vi "Create Custom Error Handler.vi"(5 "Error Description":string, 6 "T: Warning":bool, 7 "code":i32, 8 "error in":errorcluster, 10 "F: Create Error":bool=TRUE, 11 "T: Create Error":bool) -> (0 "error out":errorcluster)   [LabVIEW 2019, in "MView.lvlib"]
uses:
  Lib.llb/MView.lvlib
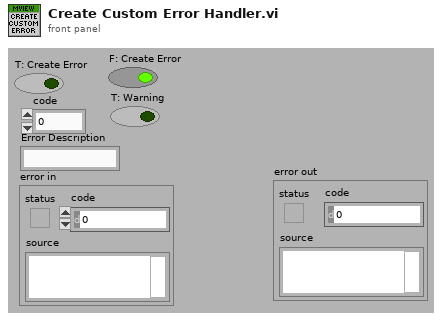
[diagram p1: front panel]
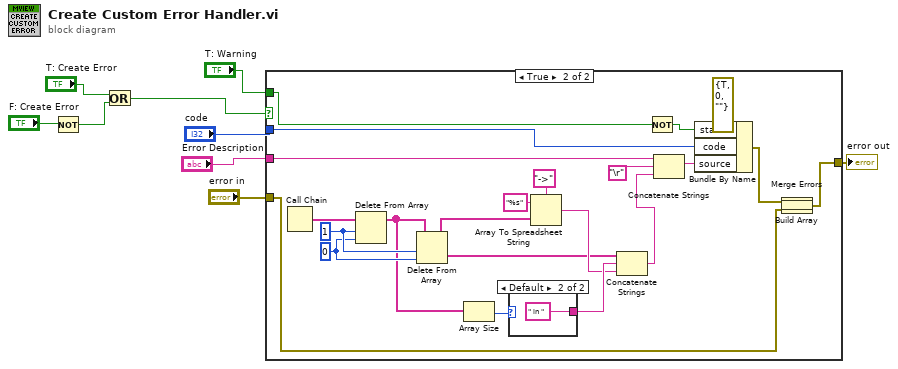
[diagram p0: block diagram]
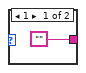
[diagram p3: hidden frame]
diagram:
  n1 = Not(x="F: Create Error") -> (.not. x?=w2:bool)
  n2 = Or(x="T: Create Error", y=w2) -> (x .or. y?=w1:bool)
  n3 = case shown="True" w1 {
    tunnel: "error in" -> [w10 w12]
    tunnel: [w10 w14] -> w6
    tunnel: "code" -> [_ w29]
    tunnel: "Error Description" -> [_ w30]
    tunnel: "T: Warning" -> [_ w15]
    frame False {
    }
    frame True {
      w22 = 0 ("Index")
      w23 = 1 ("Length")
      n4 = Call Chain() -> (call chain=w28:string[])
      n5 = Delete From Array(array=w28, length=w23, index=w22) -> (array with subset deleted=w18:string[])  [unwired: 1 out]
      n6 = Delete From Array(array=w18, length=w23, index=w22) -> (deleted portion=w19:string[], array with subset deleted=w21:string[])
      n7 = Array Size(array=w18) -> (size(s)=w20:i32)
      n8 = case shown="Default" w20 {
        tunnel: ["" " in " ("Format String")] -> w26
        frame 1 {
        }
        frame Default {
        }
      }
      n9 = Array To Spreadsheet String(delimiter (Tab)="->", array=w21, 3:"%s" ("format string")) -> (spreadsheet string=w25:string)
      n10 = Concatenate Strings(w19, w26, w25) -> (w17:string)
      n11 = Not(x=w15) -> (.not. x?=w16:bool)
      n12 = Concatenate Strings(w30, "\r", w17) -> (w32:string)
      n13 = Bundle By Name(cluster=errorcluster {"status"=TRUE, "code"=0, "source"=""} ("error out"), "status"=w16, "code"=w29, "source"=w32) -> (w13:errorcluster)
      n14 = Build Array(w13, w12) -> (w11:errorcluster[])
      n15 = Merge Errors(w11) -> (w14:errorcluster)
    }
  }
  "error out" <- w6
